vi "Delay Time.vi"(8 "error in":errorcluster, 11 "tCRD in":refnum<class "Open Path CRD.lvclass">) -> (0 "error out":errorcluster, 3 "tCRD out":refnum<class "Open Path CRD.lvclass">)   [LabVIEW 2015, in "Open Path CRD.lvclass"]
doc: "Set the delay time on the acquisition of the high frequency signal. This causes a delay after turning the laser off of x us."
uses:
  Open Path CRD.lvclass
  Open Path CRD.lvclass/Open Path CRD.ctl
  Reusable/Instrument/Instrument.lvclass/Instrument.ctl
  Accessors/Read FPGA Ref.vi
  Reusable/Instrument/Read Log Session.vi
  <vilib>/Utility/error.llb/Error Cluster From Error Code.vi
  <vilib>/rvi/errors/niLvFpgaAdjustHostInterfaceError.vi
  Open Path FPGA Ref.ctl
  <userlib>/_Session Fwk/Session - Root.lvclass
  <vilib>/rvi/interface/nirviReadWriteControl/nirviReadWriteControl.xnode
  FPGA Bitfiles/Handix_OpenPathCRD.lvbitx
  <vilib>/rvi/interface/nirviMethod/nirviMethod.xnode
  NiFpgaLv.dll
  <vilib>/rvi/errors/niLvFpgaMergeErrorWithErrorCode.vi
  Reusable/Session Log/System Log.lvclass
  <vilib>/FPGAPlugInAG/sbRIO-9637/niLvFpga_ReadFifo_sbRIO-9637.vi
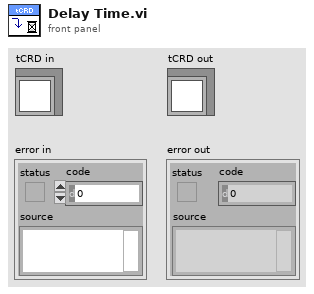
[diagram p1: front panel]
types:
  T1 = typedef "Open Path CRD.lvclass/Open Path FPGA Ref.ctl" = refnum<k20>
  T2 = typedef "Session - Root.lvclass/Session Handle.ctl" = refnum<data-value>
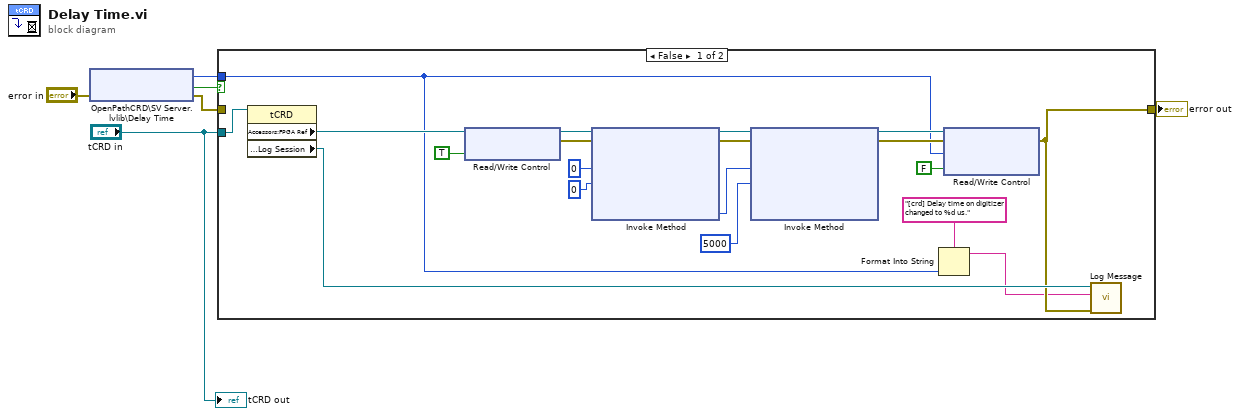
[diagram p0: block diagram]
diagram:
  n1 = shared-variable "OpenPathCRD\\SV Server.lvlib\\Delay Time"(error in="error in") -> (w4:u16, error out=w5:errorcluster, w6:bool)  [unwired: 1 in]
  n2 = case shown="False" w6 {
    tunnel: w5 -> [_ w26]
    tunnel: "tCRD in" -> [w13 _]
    tunnel: w4 -> [w8 _]
    tunnel: [w10 w26] -> w1
    frame False {
      n3 = property class="tCRD"(reference=w13) -> ("Accessors:FPGA Ref"=w12:T1, "Accessors:Log Session"=w11:T2)  [unwired: 1 in, 2 out]
      n4 = xnode "Read/Write Control"("FPGA VI Reference In"=w12, "Pause Digitizer"=TRUE) -> ("FPGA VI Reference Out"=w24:T1, "error out"=w23:errorcluster)  [unwired: 1 in]
      n5 = xnode "Invoke Method"("FPGA VI Reference In"=w24, "error in"=w23, "Number of Elements"=u32 0, "Timeout (ms)"=0) -> ("FPGA VI Reference Out"=w19:T1, "error out"=w18:errorcluster, "Elements Remaining"=w17:u32)  [unwired: 1 out]
      n6 = xnode "Invoke Method"("FPGA VI Reference In"=w19, "error in"=w18, "Number of Elements"=w17, "Timeout (ms)"=5000) -> ("FPGA VI Reference Out"=w16:T1, "error out"=w15:errorcluster)  [unwired: 2 out]
      n7 = Format Into String(format string="[crd] Delay time on digitizer changed to %d us.", w8) -> (resulting string=w7:string)  [unwired: 2 in, 1 out]
      n8 = xnode "Read/Write Control"("FPGA VI Reference In"=w16, "error in"=w15, "Delay (us)"=w8, "Pause Digitizer"=FALSE) -> ("error out"=w10:errorcluster)  [unwired: 1 out]
      n9 = call "Log Message.vi"("error in"=w10, "MSG In"=w7, "session in"=w11) -> ()  [unwired: 7 in, 2 out]
    }
    frame True {
    }
  }
  "error out" <- w1
  "tCRD out" <- "tCRD in"
